vi "Demo - Main.vi"() -> ()   [LabVIEW 2011]
uses:
  Controls/UI - All UI Objects Refs Memory - Operation.ctl
  SubVIs/UI - All UI Objects Refs Memory - Get Reference - WaveformChart.vi
panel:
  in  "Tab Control":enum32{"Page 1", "Page 2"}(tab)
  out "Cluster":cluster{"Waveform Chart":dbl}
  out "error out":errorcluster
  in  "error in":errorcluster
  in  "Stop Button":bool
  in  "Chart Visible?":bool=TRUE
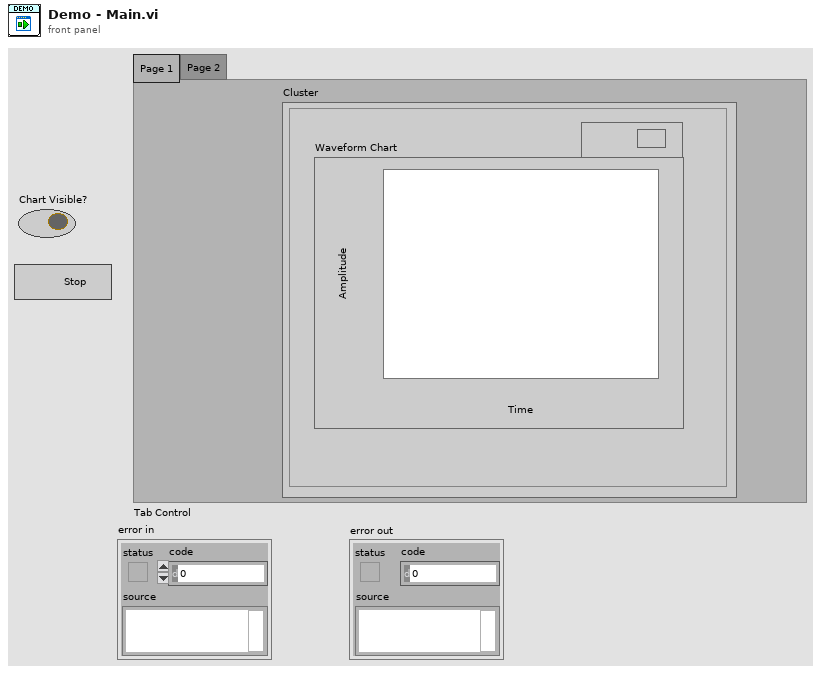
[diagram p1: front panel]
types:
  T1 = typedef "UI - All UI Objects Refs Memory - Operation.ctl" = enum16{"INIT", "GET", "ADD", "CLOSE ALL"}
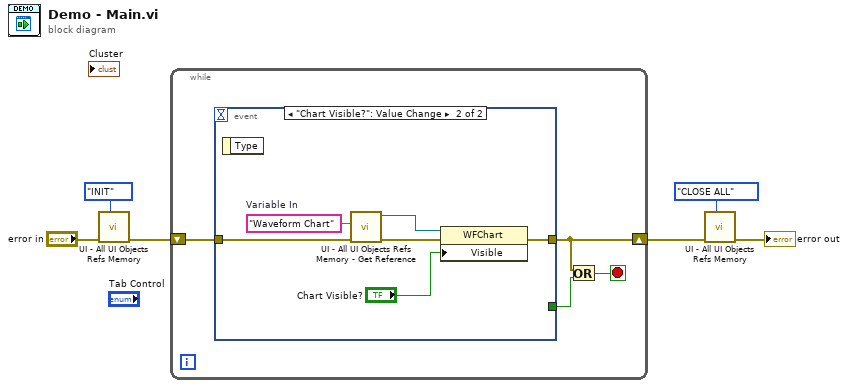
[diagram p0: block diagram]
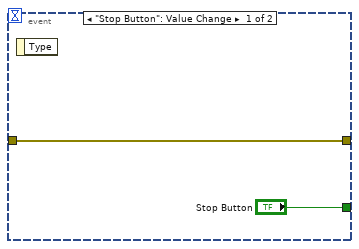
[diagram p2: hidden frame]
diagram:
  n1 = call "UI - All UI Objects Refs Memory.vi"("Operation"=UI_-_All_UI_Objects_Refs_Memory_-_Operation."INIT", "error in"="error in") -> ("error out"=w5:errorcluster)  [unwired: 8 in, 1 out]
  n2 = while {
    shift-right: [w9] -> w2
    shift-left: w5 -> [w10]
    stop <- w7 stop-if-true
    n3 = event shown="[1] \"Chart Visible?\": Value Change" {
      selector: _ -> [_ _]
      dyn-events: _ -> [_ _]
      timeout: _ -> [_ _]
      tunnel: ["Stop Button" _] -> w8
      tunnel: w10 -> [w11 w14]
      tunnel: [w11 w15] -> w9
      event "Stop Button": Value Change {
        n4 = event-data() -> ()  [unwired: 1 in, 1 out]
      }
      event "Chart Visible?": Value Change {
        w18 = "Waveform Chart"  # Variable In
        n5 = event-data() -> ()  [unwired: 1 in, 1 out]
        n6 = call-poly "UI - All UI Objects Refs Memory - Get Reference.vi"("error in (no error)"=w14, "Variable In"=w18) -> ("error out"=w16:errorcluster, "Ref Out"=w17:refnum<vi>)  [unwired: 7 in, 1 out]
        n7 = property class="WFChart"(reference=w17, error in=w16, "Visible"="Chart Visible?") -> (error out=w15:errorcluster)  [unwired: 1 out]
      }
    }
    n8 = Or(x=w9, y=w8) -> (x .or. y?=w7:bool)
  }
  n9 = call "UI - All UI Objects Refs Memory.vi"("Operation"=UI_-_All_UI_Objects_Refs_Memory_-_Operation."CLOSE ALL", "error in"=w2) -> ("error out"=→"error out":errorcluster)  [unwired: 8 in, 1 out]
